vi "子VI-查看某框-不显示界面.vi"(0 "框号":dbl format="%#_13g", 1 "框组":T4(array[cluster]), 2 "计入缺陷的Z值阈值":i32 caption="值", 3 "临界Z值":i32, 4 "计入缺陷的面积阈值":i32, 5 "临界面积百分比值":dbl, 6 "XY向分辨率":T1, 7 "缺陷灰度阈值":dbl caption="值", 8 "?":T3(plugin-control), 9 "部位信息":string[](array[string])=["", "34.500000", "32.500000", "1121", "34", "54.955926", "分层类", "不合格", ""], 10 "判定为筋条的长宽比阈值":i32, 11 "框号-更新后按顺序的值":i32) -> (20 "全部检测结果":string[][](table), 25 "flag标记簇":cluster{"框号":dbl, "数值":i32})   [LabVIEW 2018]
uses:
  <vilib>/vision/NI_Vision_Development_Module.lvlib
panel:
  out "图像Y向分辨率（mm/像素）":dbl
  out "图像X向分辨率（mm/像素）":dbl
  out "中心Y":dbl
  out "中心X":dbl
  in  "Tab Control":T2
  out "Threshold Image":T3(plugin-control)
  out "分层缺陷个数":i32
  out "合格？ 弥散类":string="fencengThreshold"
  out "合格？分层类":string="fencengThreshold"
  out "面积 (pixels)":i32
  in  "格式字符串 2":string="%f"
  in  "分隔符（'\\'代码显示）":string="\t"
  out "分层测量结果":i16[][](array[numeric])
  # "所选区域信息"
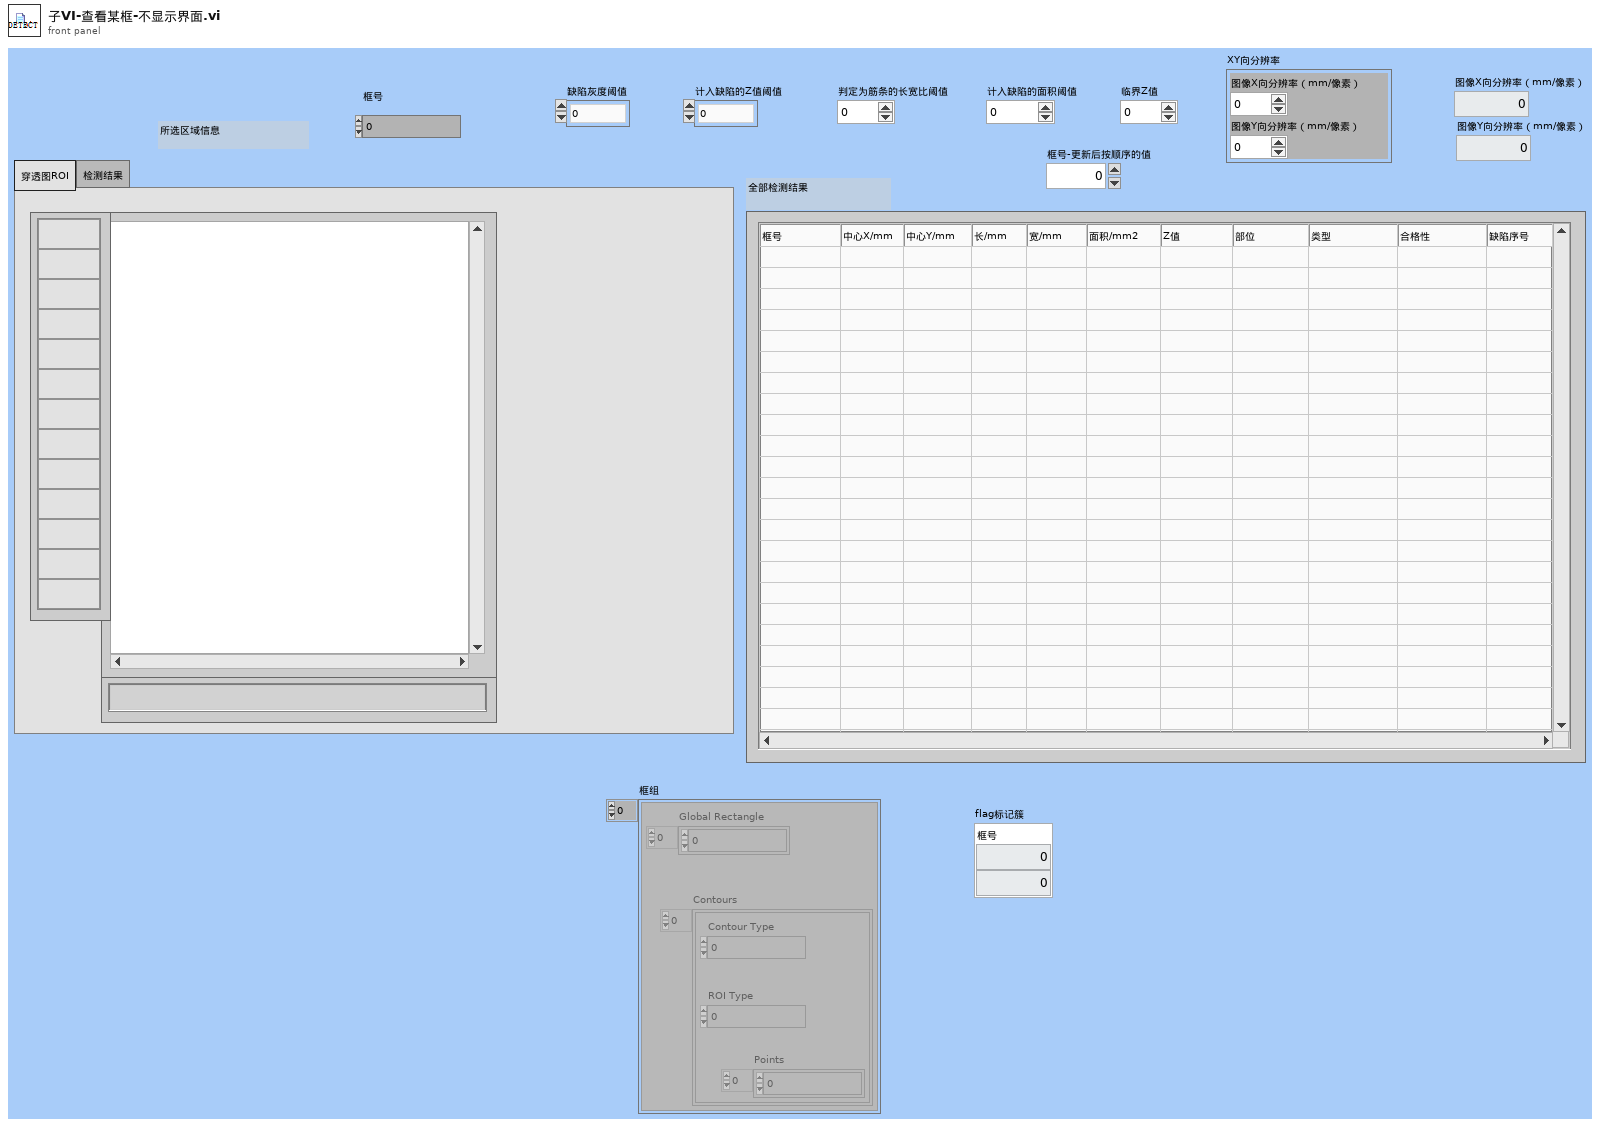
[diagram p1: front panel]
types:
  T1 = cluster{"图像X向分辨率（mm/像素）":dbl, "图像Y向分辨率（mm/像素）":dbl}
  T2 = typedef "控件2.ctl" = enum32{"穿透图ROI", "检测结果"}
  T3 = typedef "IMAQ Image.ctl" = refnum<image>
  T4 = cluster{"Global Rectangle":i32[], "Contours":cluster{"Contour Type":u32, "ROI Type":u32, "Points":i32[]}[]}[]
  T5 = typedef "Image Type" = u32
  T6 = cluster{"Global Rectangle":i32[], "Contours":cluster{"Contour Type":u32, "ROI Type":u32, "Points":i32[]}[]}
  T7 = cluster{"Desired Font (Application)":enum16{"User-specified Font", "Application Font", "System Font", "Dialog Font"}, "[User-specified Font]":cluster{"Font Name":string, "Size":i16, "Strikeout?":bool, "Italic?":bool, "Underline?":bool, "Outline?":bool, "Shadow?":bool, "Bold?":bool, "Rotation Angle":dbl}, "Horizontal Alignment":i16, "Vertical Alignment":i16}
  T8 = cluster{"histogram":u32[], "Minimal Value":sgl, "Maximal Value":sgl, "Starting Value":sgl, "Interval Width":sgl, "Mean Value":sgl, "Standard  Variation":sgl, "Area (pixels)":i32}
  T9 = typedef "Particle Parameters" = i32
  T10 = cluster{"Area":dbl, "Number of Holes":dbl, "Bounding Rect":cluster{"Left":dbl, "Top":dbl, "Right":dbl, "Bottom":dbl}, "Center of Mass":cluster{"X":dbl, "Y":dbl}, "Orientation":dbl, "Dimensions":cluster{"Width":dbl, "Height":dbl}}[]
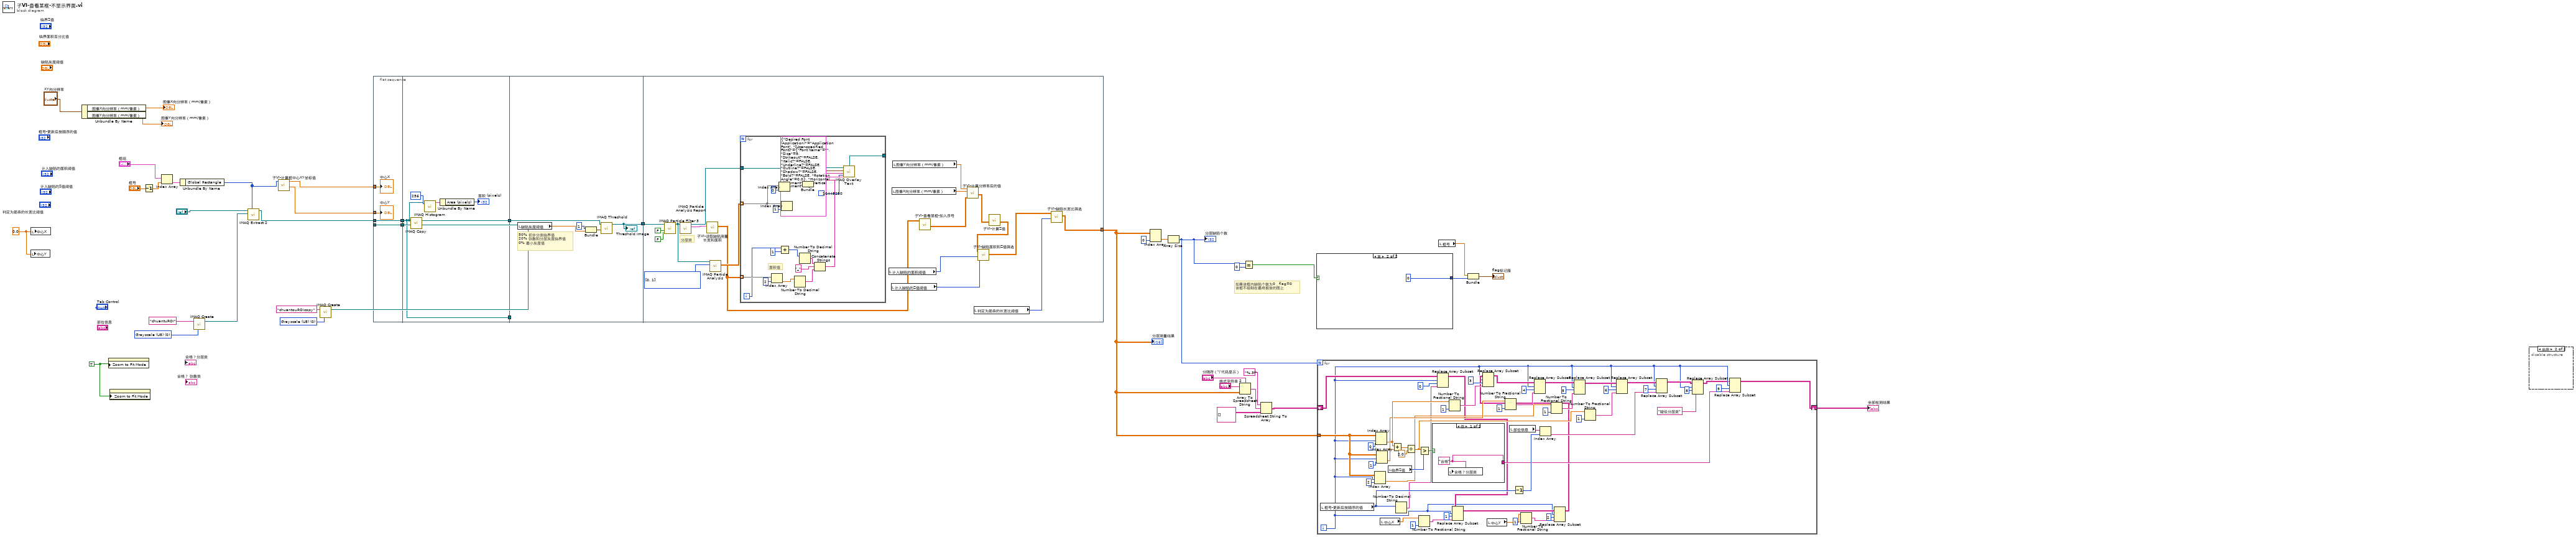
[diagram p0: block diagram]
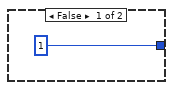
[diagram p2: hidden frame]
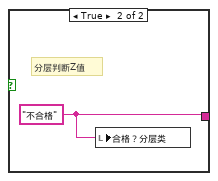
[diagram p3: hidden frame]
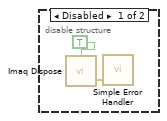
[diagram p4: hidden frame]
diagram:
  w13 = 0.0 ("中心X")
  w17 = T5 0 items=["Grayscale (U8)", "Grayscale (I16)", "Grayscale (SGL)", "Complex (CSG)", "RGB (U32)", "HSL (U32)", "RGB (U64)", "Grayscale (U16)"] ("Image Type")
  w22 = TRUE ("Zoom to Fit Mode")
  w36 = T5 0 items=["Grayscale (U8)", "Grayscale (I16)", "Grayscale (SGL)", "Complex (CSG)", "RGB (U32)", "HSL (U32)", "RGB (U64)", "Grayscale (U16)"] ("Image Type")
  # "如果该框内缺陷个数为0，flag=0\n该框不绘制在最终报告的图上"
  n1 = local write "中心Y"(w13) -> ()
  n2 = local write "中心X"(w13) -> ()
  n3 = Unbundle By Name("XY向分辨率") -> ("图像X向分辨率（mm/像素）"=→"图像X向分辨率（mm/像素）":dbl, "图像Y向分辨率（mm/像素）"=→"图像Y向分辨率（mm/像素）":dbl)
  n4 = property class="ImageControl"("Zoom to Fit Mode"=w22) -> ()  [unwired: 2 in, 2 out]
  n5 = property class="ImageControl"("Zoom to Fit Mode"=w22) -> ()  [unwired: 2 in, 2 out]
  n6 = Decrement(x="框号") -> (x-1=w38:dbl)
  n7 = Index Array(array="框组", index=w38) -> (element=w39:T6)
  n8 = Unbundle By Name(w39) -> ("Global Rectangle"=w16:i32[])
  n9 = call "IMAQ Create"("Image Name"="chuantuROI", "Image Type"=w36) -> ("New Image"=w35:T3)  [unwired: 3 in, 1 out]
  n10 = call "IMAQ Extract 2"("Optional Rectangle"=w16, "Image Dst"=w35, "Image Src"="?") -> ("Image Dst Out"=w10:T3)  [unwired: 7 in, 1 out]
  n11 = call "子VI-计算框中心XY坐标值.vi"("Global Rectangle"=w16) -> ("中心Y"=w14:dbl, "中心X"=w15:dbl)  [unwired: 9 in]
  n12 = call "IMAQ Create"("Image Name"="chuantouROIcopy", "Image Type"=w17) -> ("New Image"=w20:T3)  [unwired: 3 in, 1 out]
  n13 = flat-sequence {
    tunnel: w10 -> [w45]
    tunnel: [w45] -> w23
    tunnel: w20 -> [w44]
    tunnel: [w44] -> w19
    tunnel: w15 -> [w43]
    tunnel: w14 -> [w42]
    tunnel: [w48] -> w24
    tunnel: w23 -> [w48]
    tunnel: [w47] -> w21
    tunnel: w19 -> [w46]
    tunnel: [w56] -> w32
    tunnel: w24 -> [_]
    tunnel: w21 -> [w55]
    tunnel: [w70] -> w26
    tunnel: w32 -> [w73]
    frame #0 {
      "中心X" <- w43
      "中心Y" <- w42
    }
    frame #1 {
      n14 = call "IMAQ Copy"("Image Dst"=w46, "Image Src"=w48) -> ("Image Dst Out"=w47:T3)  [unwired: 4 in, 1 out]
      n15 = call "IMAQ Histogram"("Number of Classes"=256, "Image"=w48) -> ("Histogram Report"=w50:T8)  [unwired: 8 in, 1 out]
      n16 = Unbundle By Name(w50) -> ("Area (pixels)"=→"面积 (pixels)":i32)
    }
    frame #2 {
      # "50% 初步分类临界值\n20% 弥散和分层灰度临界值\n0% 最小灰度值"
      n17 = local read "缺陷灰度阈值"() -> (w53:dbl)
      n18 = Bundle(1, "缺陷灰度阈值"=w53) -> (w52:cluster{i32, "缺陷灰度阈值":dbl})  [unwired: 1 in]
      n19 = call "IMAQ Threshold"("Range"=w52, "Image Src"=w55) -> ("Image Dst Out"=w56:T3)  [unwired: 4 in, 5 out]
      "Threshold Image" <- w56
    }
    frame #3 {
      w66 = T9[] [0, 1] items=["Center of Mass X", "Center of Mass Y", "First Pixel X", "First Pixel Y", "Bounding Rect Left", "Bounding Rect Top", "Bounding Rect Right", "Bounding Rect Bottom", "Max Feret Diameter Start X", "Max Feret Diameter Start Y", "Max Feret Diameter End X", "Max Feret Diameter End Y", "Max Horiz. Segment Length Left", "Max Horiz. Segment Length Right", "Max Horiz. Segment Length Row", "-", "Bounding Rect Width", "Bounding Rect Height", "Bounding Rect Diagonal", "Perimeter", "Convex Hull Perimeter", "Holes' Perimeter", "Max Feret Diameter", "Equivalent Ellipse Major Axis", "Equivalent Ellipse Minor Axis", "Equivalent Ellipse Minor Axis (Feret)", "Equivalent Rect Long Side", "Equivalent Rect Short Side", "Equivalent Rect Diagonal", "Equivalent Rect Short Side (Feret)", "Average Horiz. Segment Length", "Average Vert. Segment Length", "Hydraulic Radius", "Waddel Disk Diameter", "-", "Area", "Holes' Area", "Particle & Holes' Area", "Convex Hull Area", "Image Area", "-", "Number of Holes", "Number of Horiz. Segments", "Number of Vert. Segments", "-", "Orientation", "Max Feret Diameter Orientation", "-", "% Area/Image Area", "% Area/(Particle & Holes' Area)", "Ratio of Equivalent Ellipse Axes", "Ratio of Equivalent Rect Sides", "-", "Elongation Factor", "Compactness Factor", "Heywood Circularity Factor", "Type Factor", "-", "Sum X", "Sum Y", "Sum XX", "Sum XY", "Sum YY", "Sum XXX", "Sum XXY", "Sum XYY", "Sum YYY", "-", "Moment of Inertia XX", "Moment of Inertia XY", "Moment of Inertia YY", "Moment of Inertia XXX", "Moment of Inertia XXY", "Moment of Inertia XYY", "Moment of Inertia YYY", "Norm. Moment of Inertia XX", "Norm. Moment of Inertia XY", "Norm. Moment of Inertia YY", "Norm. Moment of Inertia XXX", "Norm. Moment of Inertia XXY", "Norm. Moment of Inertia XYY", "Norm. Moment of Inertia YYY", "Hu Moment 1", "Hu Moment 2", "Hu Moment 3", "Hu Moment 4", "Hu Moment 5", "Hu Moment 6", "Hu Moment 7"] ("Pixel Measurements")
      # "分层类"
      n20 = call "IMAQ Particle Filter 3"("Image Src"=w73, "Keep/Remove Particles (F)"=FALSE, "Reject Border? (F)"=FALSE) -> ("Image Dst Out"=w65:T3)  [unwired: 10 in, 2 out]
      n21 = call "IMAQ Particle Analysis Report"("Image"=w65) -> ("Particle Reports (Pixels)"=w72:T10, "Image Out (duplicate)"=w63:T3)  [unwired: 5 in, 4 out]
      n22 = call "子VI-读取缺陷测量长宽和面积.vi"("Particle Reports (Pixels)"=w72) -> ("测量结果"=w62:dbl[][])  [unwired: 10 in]
      n23 = call "IMAQ Particle Analysis"("Pixel Measurements"=w66, "Image"=w65) -> ("Particle Measurements (Pixels)"=w64:dbl[][])  [unwired: 4 in, 5 out]
      n24 = for {
        tunnel: [w87] -> _
        tunnel: w63 -> [w95]
        tunnel: w64 -> [w92] mode=indexing
        tunnel: w62 -> [w83] mode=indexing
        i -> [w78]
        # "面积值"
        n25 = Index Array(array=w83, index=2 ("索引")) -> (element=w90:dbl)
        n26 = Index Array(array=w92, index=0 ("索引")) -> (element=w86:dbl)
        n27 = Add(x=w78, y=1) -> (x+y=w76:i32)
        n28 = Index Array(array=w92, index=1 ("索引")) -> (element=w85:dbl)
        n29 = Number To Decimal String(number=w90) -> (decimal integer string=w80:string)  [unwired: 1 in]
        n30 = Number To Decimal String(number=w76) -> (decimal integer string=w82:string)  [unwired: 1 in]
        n31 = Bundle("Numeric"=w86, "Numeric"=w85) -> (w84:cluster{"Numeric":dbl, "Numeric":dbl})  [unwired: 1 in]
        n32 = Concatenate Strings(w82, "_" ("字符串"), w80) -> (w81:string)
        n33 = call "IMAQ Overlay Text"("Text Color (black)"=u32 16448250, "Font, Size & Style"=T7 {"Desired Font (Application)"=enum."Application Font", "[User-specified Font]"={"Font Name"="", "Size"=9, "Strikeout?"=FALSE, "Italic?"=FALSE, "Underline?"=FALSE, "Outline?"=FALSE, "Shadow?"=FALSE, "Bold?"=FALSE, "Rotation Angle"=0.0}, "Horizontal Alignment"=0, "Vertical Alignment"=0}, "String"=w81, "Origin"=w84, "Image"=w95) -> ("Image Out"=w87:T3)  [unwired: 5 in, 1 out]
      }
      n34 = local read "计入缺陷的面积阈值"() -> (w71:i32)
      n35 = local read "计入缺陷的Z值阈值"() -> (w61:i32)
      n36 = local read "图像X向分辨率（mm/像素）"() -> (w68:dbl)
      n37 = local read "图像Y向分辨率（mm/像素）"() -> (w67:dbl)
      n38 = call "子VI-查看某框-加入序号.vi"("测量结果"=w62) -> ("测量结果 3"=w59:dbl[][])  [unwired: 9 in]
      n39 = call "子VI-计算分辨率后的值.vi"("测量结果"=w59, "图像X向分辨率（mm/像素）"=w68, "图像Y向分辨率（mm/像素）"=w67) -> ("初始化的数组"=w58:dbl[][])  [unwired: 7 in]
      n40 = local read "判定为筋条的长宽比阈值"() -> (w69:i32)
      n41 = call "子VI-计算Z值.vi"("分层测量结果"=w58) -> ("初始化的数组"=w57:dbl[][])  [unwired: 9 in]
      n42 = call "子VI-缺陷面积和Z值筛选.vi"("计入缺陷的Z值阈值"=w61, "计入分层缺陷的面积阈值"=w71, "分层测量结果"=w57) -> ("初始化的数组"=w60:dbl[][])  [unwired: 7 in, 1 out]
      n43 = call "子VI-缺陷长宽比筛选.vi"("判定为筋条的长宽比阈值"=w69, "分层测量结果"=w60) -> ("初始化的数组"=w70:dbl[][])  [unwired: 9 in]
    }
  }
  n44 = Index Array(array=w26, index (col)=0 ("禁用的索引 (列)")) -> (element=w34:dbl[])  [unwired: 1 in]
  n45 = Array Size(array=w34) -> (size(s)=w9:i32)
  "分层缺陷个数" <- w9
  n46 = Array To Spreadsheet String(delimiter (Tab)="分隔符（'\\'代码显示）", array=w26, 3:"格式字符串 2") -> (spreadsheet string=w29:string)
  n47 = Equal?(x=w9, y=0) -> (x = y?=w7:bool)
  n48 = Spreadsheet String To Array(format string="%.3f", spreadsheet string=w29, array type (2D Dbl)=string[][] [] ("Array")) -> (array=w25:string[][])  [unwired: 1 in]
  n49 = case shown="真" w7 {
    tunnel: [1 0] -> w5
    frame False {
    }
    frame True {
    }
  }
  n50 = for {
    N: w9 -> [_]
    tunnel: w26 -> [w104]
    shift-right: [w98] -> w12
    shift-left: w25 -> [w136]
    i -> [w102]
    n51 = local read "框号-更新后按顺序的值"() -> (w143:i32)
    n52 = Index Array(array=w104, index (row)=w102, index (col)=2 ("索引 (列)")) -> (element=w121:dbl)
    n53 = Index Array(array=w104, index (row)=w102, index (col)=0 ("禁用的索引 (列)")) -> (element=w128:dbl)
    n54 = Index Array(array=w104, index (row)=w102, index (col)=1 ("禁用的索引 (列)")) -> (element=w127:dbl)
    n55 = local read "中心X"() -> (w118:dbl)
    n56 = local read "临界Z值"() -> (w150:i32)
    n57 = Add(x=w128, y=w127) -> (x+y=w151:dbl)
    n58 = Number To Decimal String(number=w143) -> (decimal integer string=w120:string)  [unwired: 1 in]
    n59 = Divide(x=w151, y=2.0) -> (x/y=w125:dbl)
    n60 = Number To Fractional String(number=w118, precision (6)=i16 1 ("精度(6)")) -> (F-format string=w117:string)  [unwired: 2 in]
    n61 = Greater?(x=w125, y=w150) -> (0:w152:bool)
    n62 = case shown="假" w152 {
      tunnel: [w153 w154] -> w123
      frame False {
        w153 = "合格" ("合格？")
        n63 = local write "合格？分层类"(w153) -> ()
      }
      frame True {
        w154 = "不合格" ("合格？")
        # "分层判断Z值"
        n64 = local write "合格？分层类"(w154) -> ()
      }
    }
    n65 = Replace Array Subset(array=w136, new element=w120, index (row)=w102, index (col)=0 ("索引 (列)")) -> (w110:string[][])
    n66 = Number To Fractional String(number=w128, precision (6)=i16 1 ("精度(6)")) -> (F-format string=w135:string)  [unwired: 2 in]
    n67 = Replace Array Subset(array=w110, new element=w117, index (row)=w102, index (col)=1 ("索引 (列)")) -> (w111:string[][])
    n68 = local read "中心Y"() -> (w115:dbl)
    n69 = Number To Fractional String(number=w127, precision (6)=i16 1 ("精度(6)")) -> (F-format string=w134:string)  [unwired: 2 in]
    n70 = local read "部位信息"() -> (w146:string[])
    n71 = Decrement(x=w143) -> (x-1=w145:i32)
    n72 = Number To Fractional String(number=w115, precision (6)=i16 1 ("精度(6)")) -> (F-format string=w113:string)  [unwired: 2 in]
    n73 = Index Array(array=w146, index=w145) -> (element=w124:string)
    n74 = Number To Fractional String(number=w121, precision (6)=i16 1 ("精度(6)")) -> (F-format string=w131:string)  [unwired: 2 in]
    n75 = Replace Array Subset(array=w111, new element=w113, index (row)=w102, index (col)=2 ("索引 (列)")) -> (w109:string[][])
    n76 = Replace Array Subset(array=w109, new element=w135, index (row)=w102, index (col)=3 ("索引 (列)")) -> (w133:string[][])
    n77 = Replace Array Subset(array=w133, new element=w134, index (row)=w102, index (col)=4 ("索引 (列)")) -> (w132:string[][])
    n78 = Replace Array Subset(array=w132, new element=w131, index (row)=w102, index (col)=5 ("索引 (列)")) -> (w130:string[][])
    n79 = Number To Fractional String(number=w125, precision (6)=i16 1 ("精度(6)")) -> (F-format string=w126:string)  [unwired: 2 in]
    n80 = Replace Array Subset(array=w130, new element=w126, index (row)=w102, index (col)=6 ("索引 (列)")) -> (w129:string[][])
    n81 = Replace Array Subset(array=w129, new element=w124, index (row)=w102, index (col)=7 ("索引 (列)")) -> (w103:string[][])
    n82 = Replace Array Subset(array=w103, new element="疑似分层类" ("新元素/子数组"), index (row)=w102, index (col)=8 ("禁用的索引 (列)")) -> (w99:string[][])
    n83 = Replace Array Subset(array=w99, new element=w123, index (row)=w102, index (col)=9 ("索引 (列)")) -> (w98:string[][])
  }
  "全部检测结果" <- w12
  n84 = local read "框号"() -> (w6:dbl)
  n85 = Bundle("框号"=w6, w5) -> (→"flag标记簇":cluster{"框号":dbl, i32})  [unwired: 1 in]
  n86 = disable-structure shown="启用" {
    frame Disabled {
      n87 = call "Imaq Dispose"("All Images? (No)"=TRUE) -> ("error out"=w156:errorcluster)  [unwired: 5 in]
      n88 = call <vilib>:"Simple Error Handler.vi"("error in (no error)"=w156) -> ()  [unwired: 4 in, 5 out]
    }
    frame Enabled {
    }
  }
  "分层测量结果" <- w26
